vi "power_supply_choose_step.vi"(8 "error In":errorcluster, 9 "JSON string":string, 10 "Step order":string, 11 "process_ID":string) -> (0 "error IO":errorcluster)   [LabVIEW 2020]
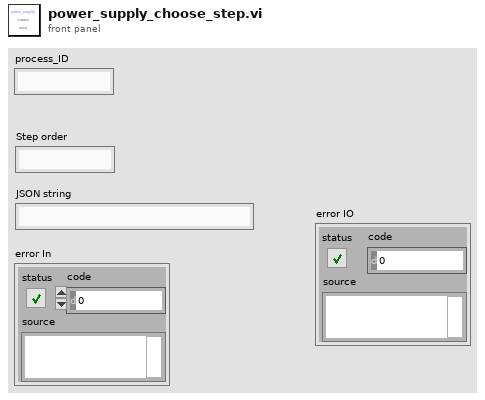
[diagram p1: front panel]
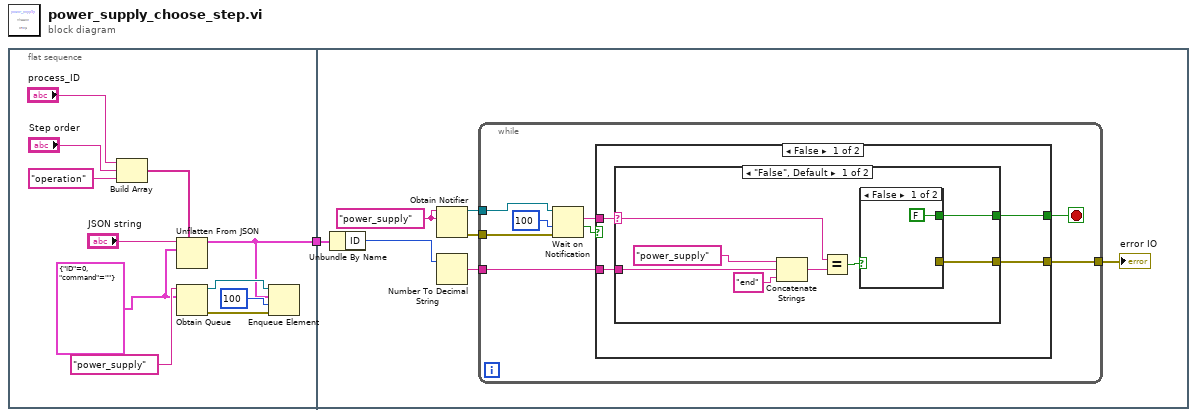
[diagram p0: block diagram]
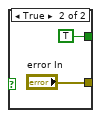
[diagram p2: hidden frame]
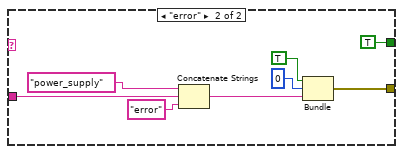
[diagram p3: hidden frame]
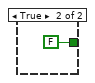
[diagram p4: hidden frame]
diagram:
  n1 = flat-sequence {
    tunnel: [w4] -> w1
    tunnel: w1 -> [w16]
    frame #0 {
      w2 = cluster{"ID":u8, "command":string} {"ID"=0, "command"=""} ("参数")
      n2 = Build Array("process_ID", "Step order", "operation" ("string")) -> (w10:string[])
      n3 = Unflatten From JSON(path=w10, JSON string="JSON string", type and defaults=w2) -> (value=w4:cluster{"ID":u8, "command":string})  [unwired: 4 in, 1 out]
      n4 = Obtain Queue(name (unnamed)="power_supply", element data type=w2) -> (queue out=w11:refnum<queue>, error out=w12:errorcluster)  [unwired: 3 in, 1 out]
      n5 = Enqueue Element(queue=w11, element=w4, timeout in ms (-1)=100, error in (no error)=w12) -> ()  [unwired: 3 out]
    }
    frame #1 {
      w17 = "power_supply" ("name (unnamed)")
      n6 = Unbundle By Name(w16) -> ("ID"=w15:u8)
      n7 = Obtain Notifier(name (unnamed)=w17, notification data type=w17) -> (notifier out=w19:refnum<notifier>, error out=w18:errorcluster)  [unwired: 2 in, 1 out]
      n8 = Number To Decimal String(number=w15) -> (decimal integer string=w13:string)  [unwired: 1 in]
      n9 = while {
        tunnel: w19 -> [w27]
        tunnel: w18 -> [w24]
        tunnel: [w21] -> w14
        tunnel: w13 -> [w20]
        stop <- w22 stop-if-true
        n10 = Wait on Notification(notifier=w27, timeout in ms (-1)=100, error in (no error)=w24) -> (notification=w23:string, timed out?=w25:bool)  [unwired: 1 in, 2 out]
        n11 = case shown="False" w25 {
          tunnel: w23 -> [w30 _]
          tunnel: [w31 FALSE] -> w22
          tunnel: [w29 _] -> w21
          tunnel: w20 -> [w28 _]
          frame False {
            n12 = case shown="\"False\", Default" w30 {
              selector: w30 -> [w37 _]
              tunnel: [w38 TRUE] -> w31
              tunnel: [w32 w47] -> w29
              tunnel: w28 -> [w33 w46]
              frame "False", Default {
                n13 = Concatenate Strings("power_supply" ("string"), w33, "end" ("string")) -> (w35:string)
                n14 = Equal?(x=w37, y=w35) -> (x = y?=w39:bool)
                n15 = case shown="False" w39 {
                  tunnel: [FALSE TRUE] -> w38
                  tunnel: [_ "error In"] -> w32
                  frame False {
                  }
                  frame True {
                  }
                }
              }
              frame "error" {
                n16 = Concatenate Strings("power_supply" ("string"), w46, "error" ("string")) -> (w44:string)
                n17 = Bundle("status"=TRUE, "code"=0, w44) -> (w47:cluster{"status":bool, "code":i32, string})  [unwired: 1 in]
              }
            }
          }
          frame True {
          }
        }
      }
      "error IO" <- w14
    }
  }
